vi "Get Command Description.vi"(0 "SLSC Local in":refnum<class "SLSC Local.lvclass">, 5 "command in":refnum<k21>, 11 "error in (no error)":errorcluster) -> (4 "SLSC Local out":refnum<class "SLSC Local.lvclass">, 6 "command out":refnum<k21>, 10 "Cmd.Descr":string, 15 "error out":errorcluster)   [LabVIEW 2015, in "SLSC Local.lvclass"]
uses:
  SLSC Local.lvclass
  <resource>/objmgr/slsc.rc
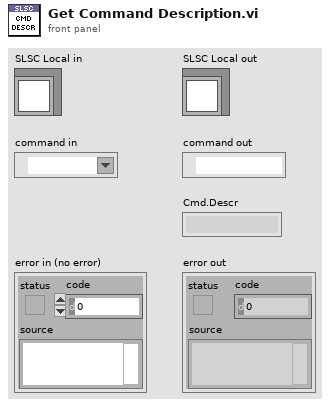
[diagram p1: front panel]
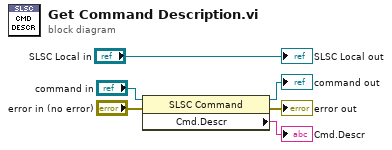
[diagram p0: block diagram]
diagram:
  n1 = property class="SLSC Command"(reference="command in", error in="error in (no error)") -> (reference out=→"command out":refnum<k21>, error out=→"error out":errorcluster, "Cmd.Descr"=→"Cmd.Descr":string)
  "SLSC Local out" <- "SLSC Local in"
